vi "TCP Fast Listen.vi"(6 "TCP_NODELAY (true)":bool, 7 "net address":u32, 8 "error in (no error)":errorcluster, 9 "timeout ms (wait forever: -1)":i32=-1, 10 "port":u16) -> (0 "error out":errorcluster, 1 "remote port":u16, 2 "remote address":string, 3 "connection ID":refnum<k5>)   [LabVIEW 2020]
doc: "Creates a listener and waits for an accepted TCP network connection at the specified <B>port</B>. This is a custom version of <B>TCP Listen</B> modified to reduce connection time by not resolving the connecting hostname. Also, disables the Nagel algorithm to improve latency in query/response applications."
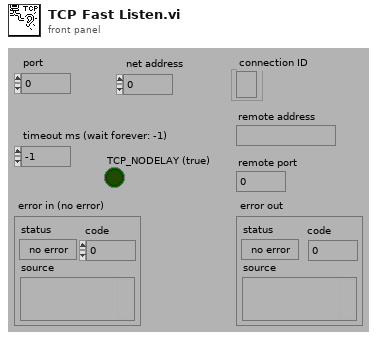
[diagram p1: front panel]
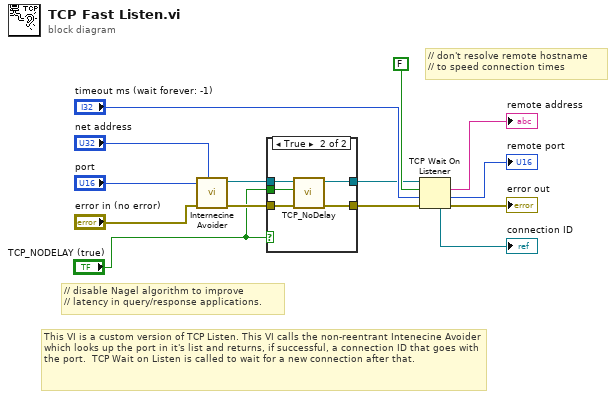
[diagram p0: block diagram]
diagram:
  # "// disable Nagel algorithm to improve\n// latency in query/response applications."
  # "// don't resolve remote hostname\n// to speed connection times"
  # "This VI is a custom version of TCP Listen. This VI calls the non-reentrant Intenecine Avoider which looks up the port in it's list and returns, if successful, a connection ID that goes with the port.  TCP Wait on Listen is called to wait for a new connection after that."
  n1 = call <vilib>:"Internecine Avoider.vi"("net address"="net address", "error in"="error in (no error)", "port"="port") -> ("error out"=w3:errorcluster, "connection ID"=w5:refnum<k5>)  [unwired: 7 in]
  n2 = case shown="True" "TCP_NODELAY (true)" {
    tunnel: w5 -> [w16 w21]
    tunnel: [w16 w20] -> w4
    tunnel: w3 -> [w15 w19]
    tunnel: [w15 w18] -> w2
    tunnel: "TCP_NODELAY (true)" -> [_ w17]
    frame False {
    }
    frame True {
      n3 = call "TCP_NoDelay.vi"("error in (no error)"=w19, "TCP_NODELAY (true)"=w17, "connID"=w21) -> ("error out"=w18:errorcluster, "connID 2"=w20:refnum<k5>)  [unwired: 3 in]
    }
  }
  n4 = TCP Wait On Listener(8:w2, 9:"timeout ms (wait forever: -1)", 10:FALSE ("resolve remote address (T)"), 11:w4) -> (0:→"error out":errorcluster, 1:→"remote port":u16, 2:→"remote address":string, 4:→"connection ID":refnum<k5>)  [unwired: 1 out]
